vi "CheckBug.vi"() -> ()   [LabVIEW 2017]
panel:
  out "last row":i32[](array[numeric])
  out "size(s)":i32[](array[numeric])
  out "time size":i32
  out "data size":i32
  out "cycle #":i32
  out "XY Graph":cluster{timestamp[], i32[]}[](graph)
  out "appended array":i32[][](array[numeric])
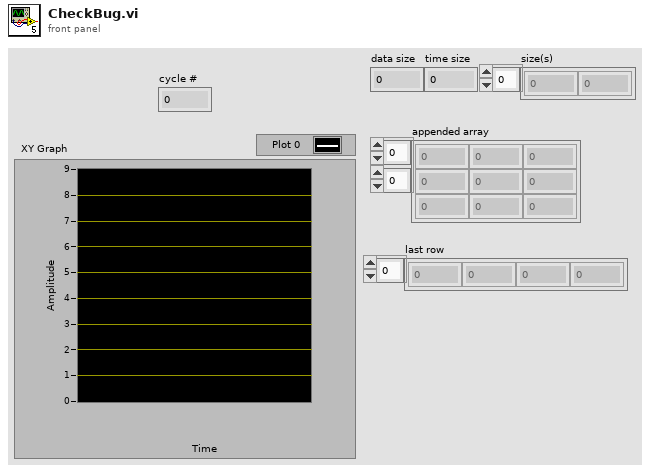
[diagram p1: front panel]
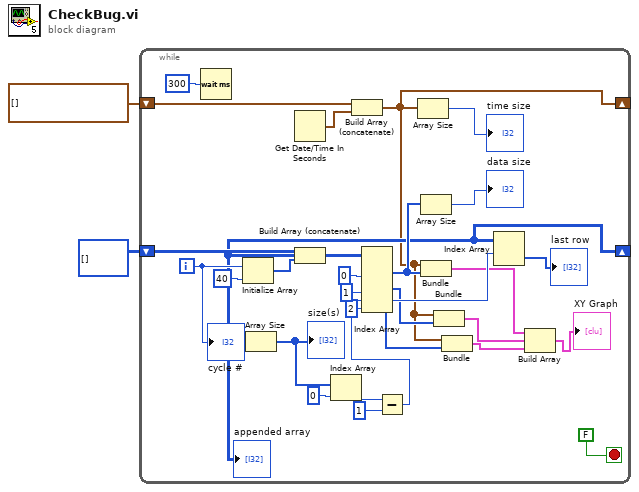
[diagram p0: block diagram]
diagram:
  n1 = while {
    shift-right: [w18] -> _
    shift-left: i32[][] [] -> [w19]
    shift-right: [w8] -> _
    shift-left: timestamp[] [] -> [w25]
    i -> [w29]
    stop <- FALSE stop-if-true
    n2 = Wait (ms)(milliseconds to wait=u32 300) -> ()  [unwired: 1 out]
    n3 = Initialize Array(w29, 40 ("dimension size")) -> (w27:i32[])
    n4 = Get Date/Time In Seconds() -> (seconds since 1Jan1904=w26:timestamp)
    n5 = Build Array (concatenate)(w19, w27) -> (w18:i32[][])
    "appended array" <- w18
    n6 = Array Size(array=w18) -> (size(s)=w17:i32[])
    "size(s)" <- w17
    n7 = Index Array(array=w17, index=0) -> (element=w14:i32)
    n8 = Build Array (concatenate)(w25, w26) -> (w8:timestamp[])
    n9 = Index Array(array=w18, index (col) #1=0 ("disabled index (col)"), index (col) #2=1 ("index (col)"), index (col) #3=2 ("index (col)")) -> (element #1=w23:i32[], element #2=w9:i32[], element #3=w7:i32[])  [unwired: 3 in]
    n10 = Subtract(x=w14, y=1) -> (x-y=w12:i32)
    n11 = Array Size(array=w8) -> (size(s)=→"time size":i32)
    n12 = Array Size(array=w23) -> (size(s)=→"data size":i32)
    n13 = Bundle(w8, w23) -> (w6:cluster{timestamp[], i32[]})  [unwired: 1 in]
    n14 = Bundle(w8, w9) -> (w5:cluster{timestamp[], i32[]})  [unwired: 1 in]
    n15 = Bundle(w8, w7) -> (w4:cluster{timestamp[], i32[]})  [unwired: 1 in]
    n16 = Index Array(array=w18, index (row)=w12) -> (element=→"last row":i32[])  [unwired: 1 in]
    n17 = Build Array(w6, w5, w4) -> (→"XY Graph":cluster{timestamp[], i32[]}[])
    "cycle #" <- w29
  }
